vi "TESTBENCH_Menu.vi"() -> ()   [LabVIEW 2019]
doc: "JSMA Module Template - Top Level UI 0.2.0.4\nRob Humfeld - Jet Engineering\nCopyright (c) 2019, Jet Engineering"
uses:
  Menu Button.xctl
panel:
  out "Ok?":bool
  out "Level":string
  out "Button Pressed":string
  in  "stop":bool
  in  "Menu Button":T1(xcontrol)
  out "MenuConfig":variant
  in  "Configuration Path":path=path "C:/Projects/Trackside-CrawlerFinalDriveTestStand/Codeline/Main Codeline/Software/Config Files_Host/MenuConfig.ini"
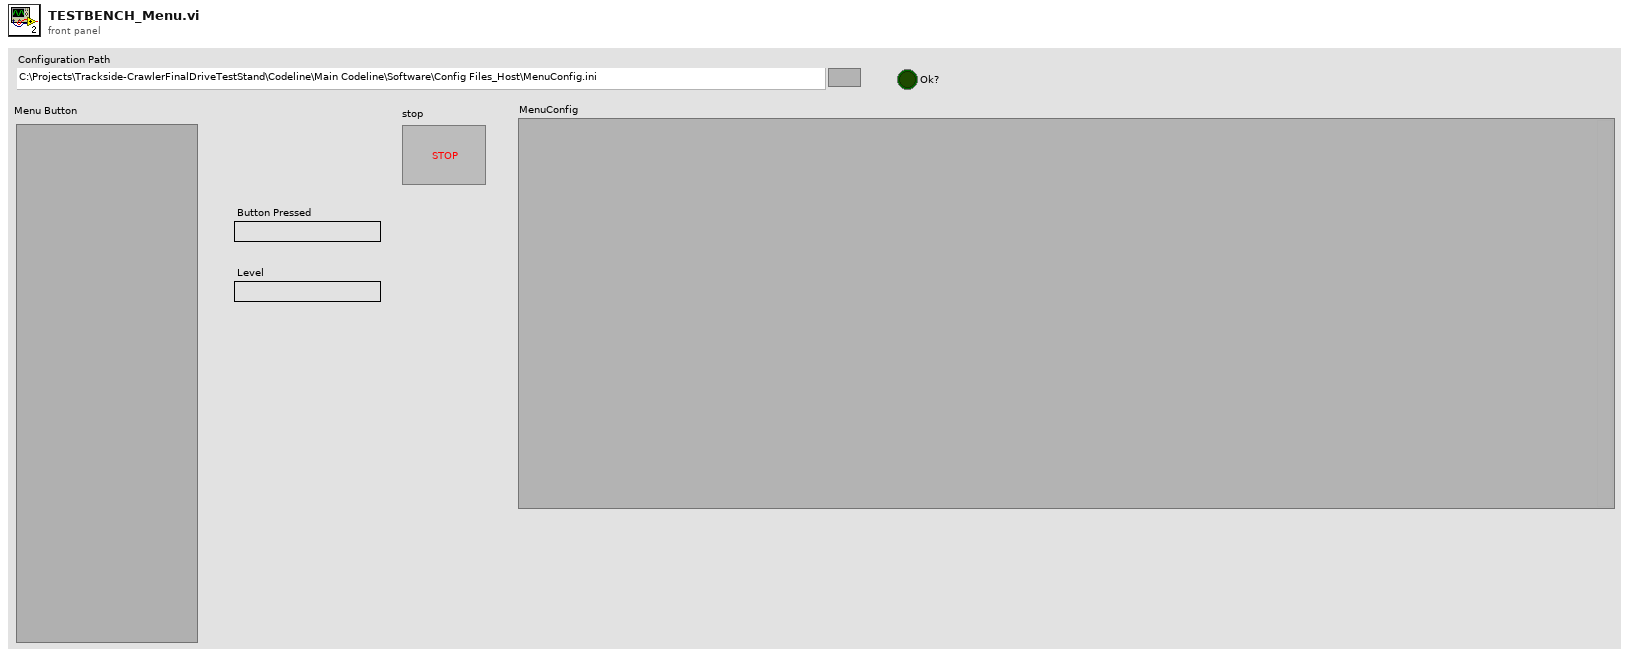
[diagram p1: front panel]
types:
  T1 = cluster{"Button Pressed":string, "Level":string, "Menu Config":variant}
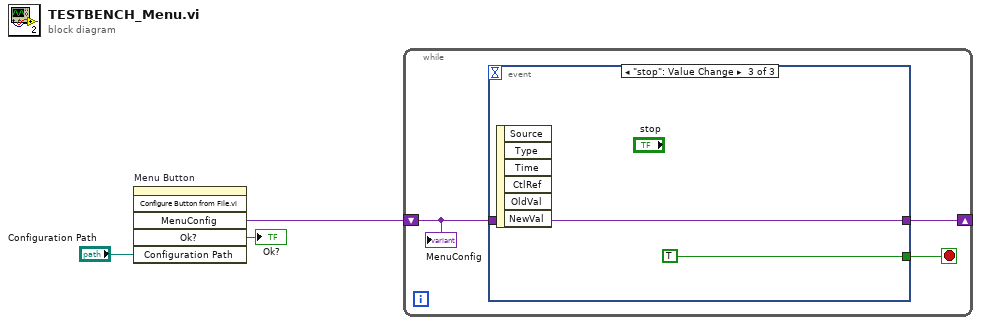
[diagram p0: block diagram]
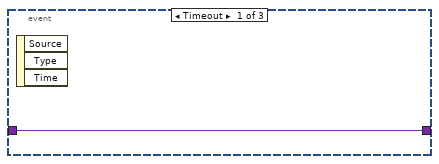
[diagram p2: hidden frame]
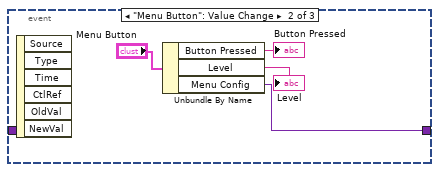
[diagram p3: hidden frame]
diagram:
  n1 = invoke on="Menu Button" class="Menu Button (strict)" method="Configure Button from File.vi"("Configuration Path"="Configuration Path") -> ("MenuConfig"=w2:variant, "Ok?"=→"Ok?":bool)  [unwired: 5 in, 4 out]
  n2 = while {
    shift-right: [w5] -> _
    shift-left: w2 -> [w4]
    stop <- w6 stop-if-true
    n3 = event shown="[2] \"stop\": Value Change" {
      selector: _ -> [_ _ _]
      dyn-events: _ -> [_ _ _]
      timeout: _ -> [_ _ _]
      tunnel: [_ _ TRUE] -> w6
      tunnel: [w7 w8 w12] -> w5
      tunnel: w4 -> [w7 _ w12]
      event Timeout {
        n4 = event-data() -> ()  [unwired: 1 in, 3 out]
      }
      event "Menu Button": Value Change {
        n5 = event-data() -> ()  [unwired: 1 in, 6 out]
        n6 = Unbundle By Name("Menu Button") -> ("Button Pressed"=→"Button Pressed":string, "Level"=→"Level":string, "Menu Config"=w8:variant)
      }
      event "stop": Value Change {
        n7 = event-data() -> ()  [unwired: 1 in, 6 out]
      }
    }
    "MenuConfig" <- w4
  }
